vi "ActionVIOnCompile.vi"(8 "error in":errorcluster, 11 "Device Item Ref in":T1 format="%.0x") -> (0 "error out":errorcluster)   [LabVIEW 2020, in "Ballard ARINC 429 System Explorer.lvlib"]
uses:
  Ballard ARINC 429 System Explorer.lvlib
  <vilib>/NI VeriStand/Custom Device API/Custom Device Item Ref.ctl
  Shared/Compiled.Settings.ctl
  Shared/Inline Execution Unit Compiled Information.ctl
  <vilib>/NI VeriStand/Custom Device API/Data Reference.ctl
  <vilib>/NI VeriStand/Custom Device API/Block Data Reference.ctl
  Shared/Asynchronous Execution Unit Compiled Information.ctl
  Includes/Ballard ARINC 429 Engine.lvlibp/Custom Device Support/Engine/Interfaces/Execution Unit Factory/Execution Unit Factory.lvclass
  Includes/Ballard ARINC 429 Engine.lvlibp/Custom Device Support/Engine/Implementation/Execution Unit Factory/Execution Unit Factory.lvclass
  C:/Git/niveristand-ballard-arinc429-custom-device/Includes/Ballard ARINC 429 Engine.lvlibp/Custom Device Support/Engine/Interfaces/Execution Unit Factory/Execution Unit Factory.lvclass
  Custom Device Support/Scripting/Constants.vi
  <vilib>/NI VeriStand/Custom Device API/Set Item Property (Variant).vi
  <vilib>/NI VeriStand/Custom Device API/Custom Device API.lvlib
  Shared/Ballard ARINC 429 Shared.lvlib
  Custom Device Support/Scripting/Ballard ARINC 429 Scripting.lvlib
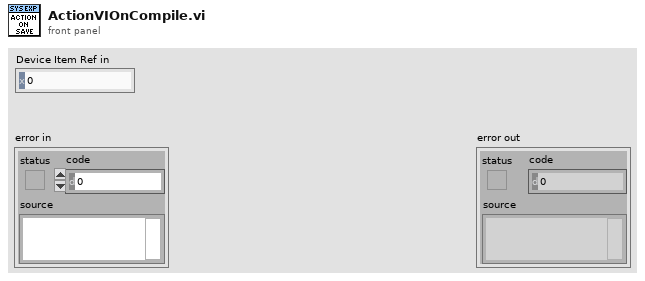
[diagram p1: front panel]
types:
  T1 = typedef "Custom Device API.lvlib/Custom Device Item Ref.ctl" = u64
  T2 = typedef "Ballard ARINC 429 Shared.lvlib/Compiled.Settings.ctl" = cluster{"Name":string, "Inline Execution Unit Compiled Information":T3[], "Asynchronous Execution Unit Compiled Information":T6[]}
  T3 = typedef "Ballard ARINC 429 Shared.lvlib/Inline Execution Unit Compiled Information.ctl" = cluster{"Flattened Execution Unit":string, "Incoming Buffer":dbl[], "Outgoing Buffer":dbl[], "Incoming Data References":T4[], "Outgoing Data References":T5[]}
  T4 = typedef "Custom Device API.lvlib/Data Reference.ctl" = i32
  T5 = typedef "Custom Device API.lvlib/Block Data Reference.ctl" = cluster{"Data Reference":T4, "Offset":u64, "Length":u64}
  T6 = typedef "Ballard ARINC 429 Shared.lvlib/Asynchronous Execution Unit Compiled Information.ctl" = cluster{"Flattened Execution Unit":string, "Incoming Channel Group Name":string, "Outgoing Channel Group Name":string}
  T7 = typedef "Custom Device API.lvlib/Custom Device Item Info.ctl" = cluster{"Name":string, "Is Channel":bool, "GUID":string, "Is Waveform":bool}
  T8 = typedef "Ballard ARINC 429 Engine.lvlibp/Interfaces.lvlib/Execution Unit Information.ctl" = cluster{"Execution Unit":refnum<class "Execution Unit.lvclass">, "Incoming Channels":T9[], "Outgoing Channels":T9[]}
  T9 = typedef "Ballard ARINC 429 Engine.lvlibp/Custom Device API.lvlib/Custom Device Item Ref.ctl" = u64
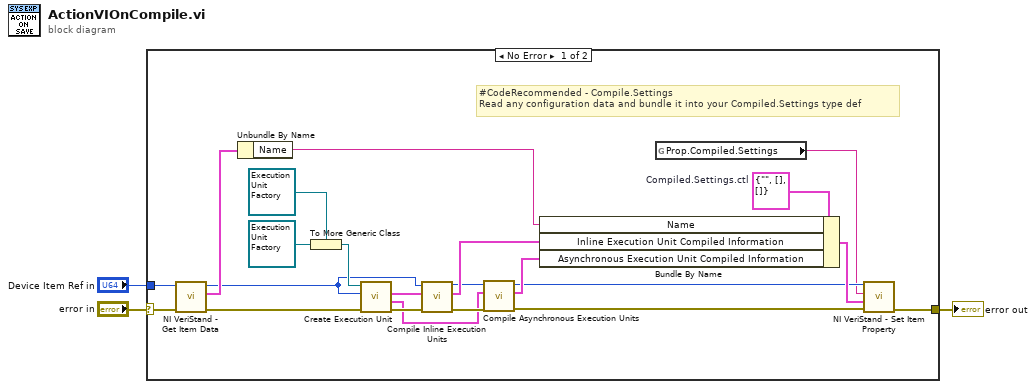
[diagram p0: block diagram]
diagram:
  n1 = case shown="No Error" "error in" {
    selector: "error in" -> [w21 w26]
    tunnel: [w24 w26] -> w2
    tunnel: "Device Item Ref in" -> [w18 _]
    frame No Error {
      w22 = T2 {"Name"="", "Inline Execution Unit Compiled Information"=[], "Asynchronous Execution Unit Compiled Information"=[]}  # Compiled.Settings.ctl
      # "#CodeRecommended - Compile.Settings\nRead any configuration data and bundle it into your Compiled.Settings type def"
      n2 = call <vilib>:"NI VeriStand - Get Item Data.vi"("error in (no error)"=w21, "Item Ref in"=w18) -> ("error out"=w10:errorcluster, "Item Info"=w23:T7, "Item Ref out"=w9:T1)  [unwired: 6 in, 1 out]
      n3 = Unbundle By Name(w23) -> ("Name"=w19:string)
      n4 = To More Generic Class(target class=refnum<class "Execution Unit Factory.lvclass"> refnum ("Communication Bus Template Interfaces:Interfaces.lvlib:Execution Unit Factory.lvclass"), reference=refnum<class "Execution Unit Factory.lvclass"> refnum ("Communication Bus Template Interfaces:Implementation.lvlib:Execution Unit Factory.lvclass")) -> (generic class reference=w17:refnum<class "Execution Unit Factory.lvclass">)
      n5 = call-dynamic "Create Execution Unit.vi"("error in"=w10, "Item Ref"=w9, "Execution Unit Factory in"=w17) -> ("error out"=w20:errorcluster, "Asynchronous Execution Units"=w7:T8[], "Inline Execution Units"=w15:T8[])  [unwired: 5 in, 1 out]
      n6 = call "Compile Inline Execution Units.vi"("error in"=w20, "Inline Execution Units"=w15, "Device Ref in"=w9) -> ("error out"=w14:errorcluster, "Compiled Inline Execution Units"=w16:T3[], "Device Ref out"=w13:T1)  [unwired: 6 in]
      n7 = call "Compile Asynchronous Execution Units.vi"("Device Ref in"=w13, "Asynchronous Execution Units"=w7, "error in"=w14) -> ("Device Ref out"=w8:T1, "Compiled Asynchronous Execution Units"=w12:T6[], "error out"=w11:errorcluster)  [unwired: 5 in]
      n8 = Bundle By Name(cluster=w22, "Name"=w19, "Inline Execution Unit Compiled Information"=w16, "Asynchronous Execution Unit Compiled Information"=w12) -> (w25:T2)
      n9 = global read "Constants.vi" "Prop.Compiled.Settings"() -> (w4:string)
      n10 = call-poly <vilib>:"NI VeriStand - Set Item Property.vi"("error in (no error)"=w11, "Value"=w25, "Property Name"=w4, "Item Ref in"=w8) -> ("error out"=w24:errorcluster)  [unwired: 5 in, 2 out]
    }
    frame Error {
    }
  }
  "error out" <- w2
